vi "Teleop.vi"(10 "Match Info":T1={"Autonomous Elapsed Seconds"=0.0, "TeleOp Elapsed Seconds"=0.0, "Disabled Elapsed Seconds"=0.0, "Visited Autonomous"=FALSE, "Visited TeleOp"=FALSE, "Visited Disabled"=FALSE, "Autonomous Settings"={"Autonomous Style"=enum."Independent", "VI Refnum"=refnum}}, 11 "Call Context":T2) -> ()   [LabVIEW 2019]
doc: "This VI is called for each TeleOp packet received from the DS where the robot is not disabled. It is often used to read from the joysticks and update I/O or to update setpoints for timed control loops. It should complete and return within 20 milliseconds or it may miss DS packets."
uses:
  <vilib>/Rock Robotics/WPI/DriverStation/WPI_DriverStationDerivedRobotMode.ctl
  <vilib>/Rock Robotics/WPI/DriverStation/WPI_DriverStationMatch Info.ctl
  <vilib>/Rock Robotics/WPI/ThirdParty/Phoenix-LabVIEW/Motor Controller/Controls/CTRE_Phoenix_MotorControl_ControlMode.ctl
  <vilib>/Rock Robotics/WPI/Utilities/WPI_GetSetVariantRefNum.vi
  <vilib>/Rock Robotics/WPI/ThirdParty/Phoenix-LabVIEW/Motor Controller/Get/CTRE_Phoenix_MotorController_GetSelectedSensorData.vi
  <vilib>/Rock Robotics/WPI/ThirdParty/Phoenix-LabVIEW/Motor Controller/Get/CTRE_Phoenix_MotorController_GetSupplyAndStatorCurrent_Enhanced.vi
  <vilib>/Rock Robotics/WPI/ThirdParty/Phoenix-LabVIEW/Motor Controller/Get/CTRE_Phoenix_MotorController_GetVoltage.vi
  <vilib>/Rock Robotics/WPI/ThirdParty/Phoenix-LabVIEW/Motor Controller/Get/CTRE_Phoenix_MotorController_IntegratedSensorData_TalonFX.vi
panel:
  out "Waveform Chart":cluster{dbl, "Velocity":dbl}(graph)
  out "RPM":dbl
  out "Velocity (Raw Sensor Units per 100 ms)":i32
  out "Stator Current":dbl
  out "Supply Current":dbl
  out "Joystick Y axis":dbl
  in  "Reverse Peak Percent Output":dbl=-1.0
  in  "Forward Peak Percent Output":dbl=1.0
  out "Output Voltage":dbl
  out "Absolute Position":dbl
  out "Percent Voltage":dbl
  out "Velocity":dbl format="%.2f"
  out "Position":dbl
  # "INFORMATION"
  # "CONTROLS"
  # "FALCON 500 INFORMATION AND CONTROLS"
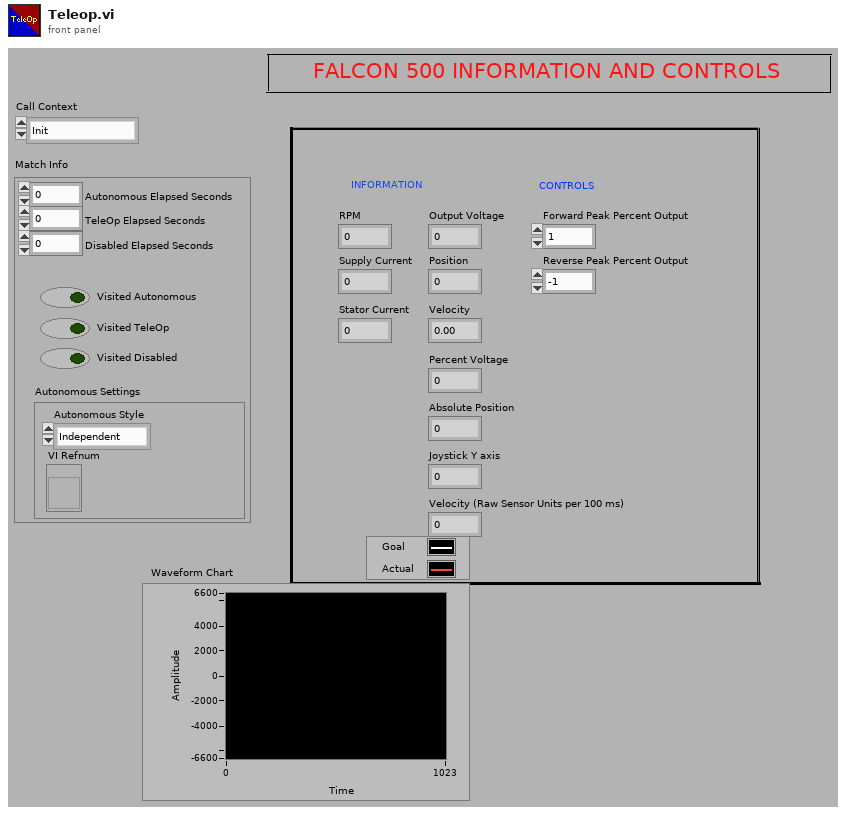
[diagram p1: front panel]
types:
  T1 = typedef "WPI_DriverStationMatch Info.ctl" = cluster{"Autonomous Elapsed Seconds":dbl, "TeleOp Elapsed Seconds":dbl, "Disabled Elapsed Seconds":dbl, "Visited Autonomous":bool, "Visited TeleOp":bool, "Visited Disabled":bool, "Autonomous Settings":cluster{"Autonomous Style":enum16{"Iterative", "Independent"}, "VI Refnum":refnum<vi>}}
  T2 = typedef "WPI_DriverStationDerivedRobotMode.ctl" = enum16{"Init", "Execute", "Stop"}
  T3 = typedef "CTRE_Phoenix_MotorControl_ControlMode.ctl" = u16
  T4 = typedef "WPI_JoystickDevRef.ctl" = cluster{"Device":T5}
  T5 = typedef "WPI_JoystickDeviceEnum.ctl" = enum16{"USB 0", "USB 1", "USB 2", "USB 3", "USB 4", "USB 5"}
  T6 = typedef "WPI_MotorControlDeviceRef.ctl" = cluster{"DeviceStatus":errorcluster, "Type":T7, "PWM":cluster{"PWM Channel":T8, "DeadBand":T9}, "CAN":cluster{"Device Number":u8, "SetOutput VI Ref":variant, "GetOutput VI Ref":variant, "Enable VI Ref":variant, "Disable VI Ref":variant, "Data":variant}, "Invert":bool, "DIO PWM":cluster{"PWM \"Enable\" Channel":T8, "DIOChannel":T10, "PWM Rate":dbl}}
  T7 = typedef "WPI_MotorControlType.ctl" = enum16{"PWM", "CAN", "DIO PWM"}
  T8 = typedef "FPGA_DIOPWMChannel.ctl" = enum8{"PWM 0", "PWM 1", "PWM 2", "PWM 3", "PWM 4", "PWM 5", "PWM 6", "PWM 7", "PWM 8", "PWM 9", "PWM MXP 0", "PWM MXP 1", "PWM MXP 2", "PWM MXP 3", "PWM MXP 4", "PWM MXP 5", "PWM MXP 6", "PWM MXP 7", "PWM MXP 8", "PWM MXP 9", "Invalid"}
  T9 = typedef "WPI_PWMDeadband.ctl" = cluster{"Name":string, "maxPositivePwm":i32, "minPositivePwm":i32, "centerPwm":i32, "maxNegativePwm":i32, "minNegativePwm":i32, "angularRange":u16}
  T10 = typedef "FPGA_DIOChannel.ctl" = enum8{"DIO 0", "DIO 1", "DIO 2", "DIO 3", "DIO 4", "DIO 5", "DIO 6", "DIO 7", "DIO 8", "DIO 9", "DIO MXP 0", "DIO MXP 1", "DIO MXP 2", "DIO MXP 3", "DIO MXP 4", "DIO MXP 5", "DIO MXP 6", "DIO MXP 7", "DIO MXP 8", "DIO MXP 9", "DIO MXP 10", "DIO MXP 11", "DIO MXP 12", "DIO MXP 13", "DIO MXP 14", "DIO MXP 15", "SPI Port CS1", "SPI Port CS2", "SPI Port CS3", "SPI Port MISO", "SPI Port MOSI", "Invalid"}
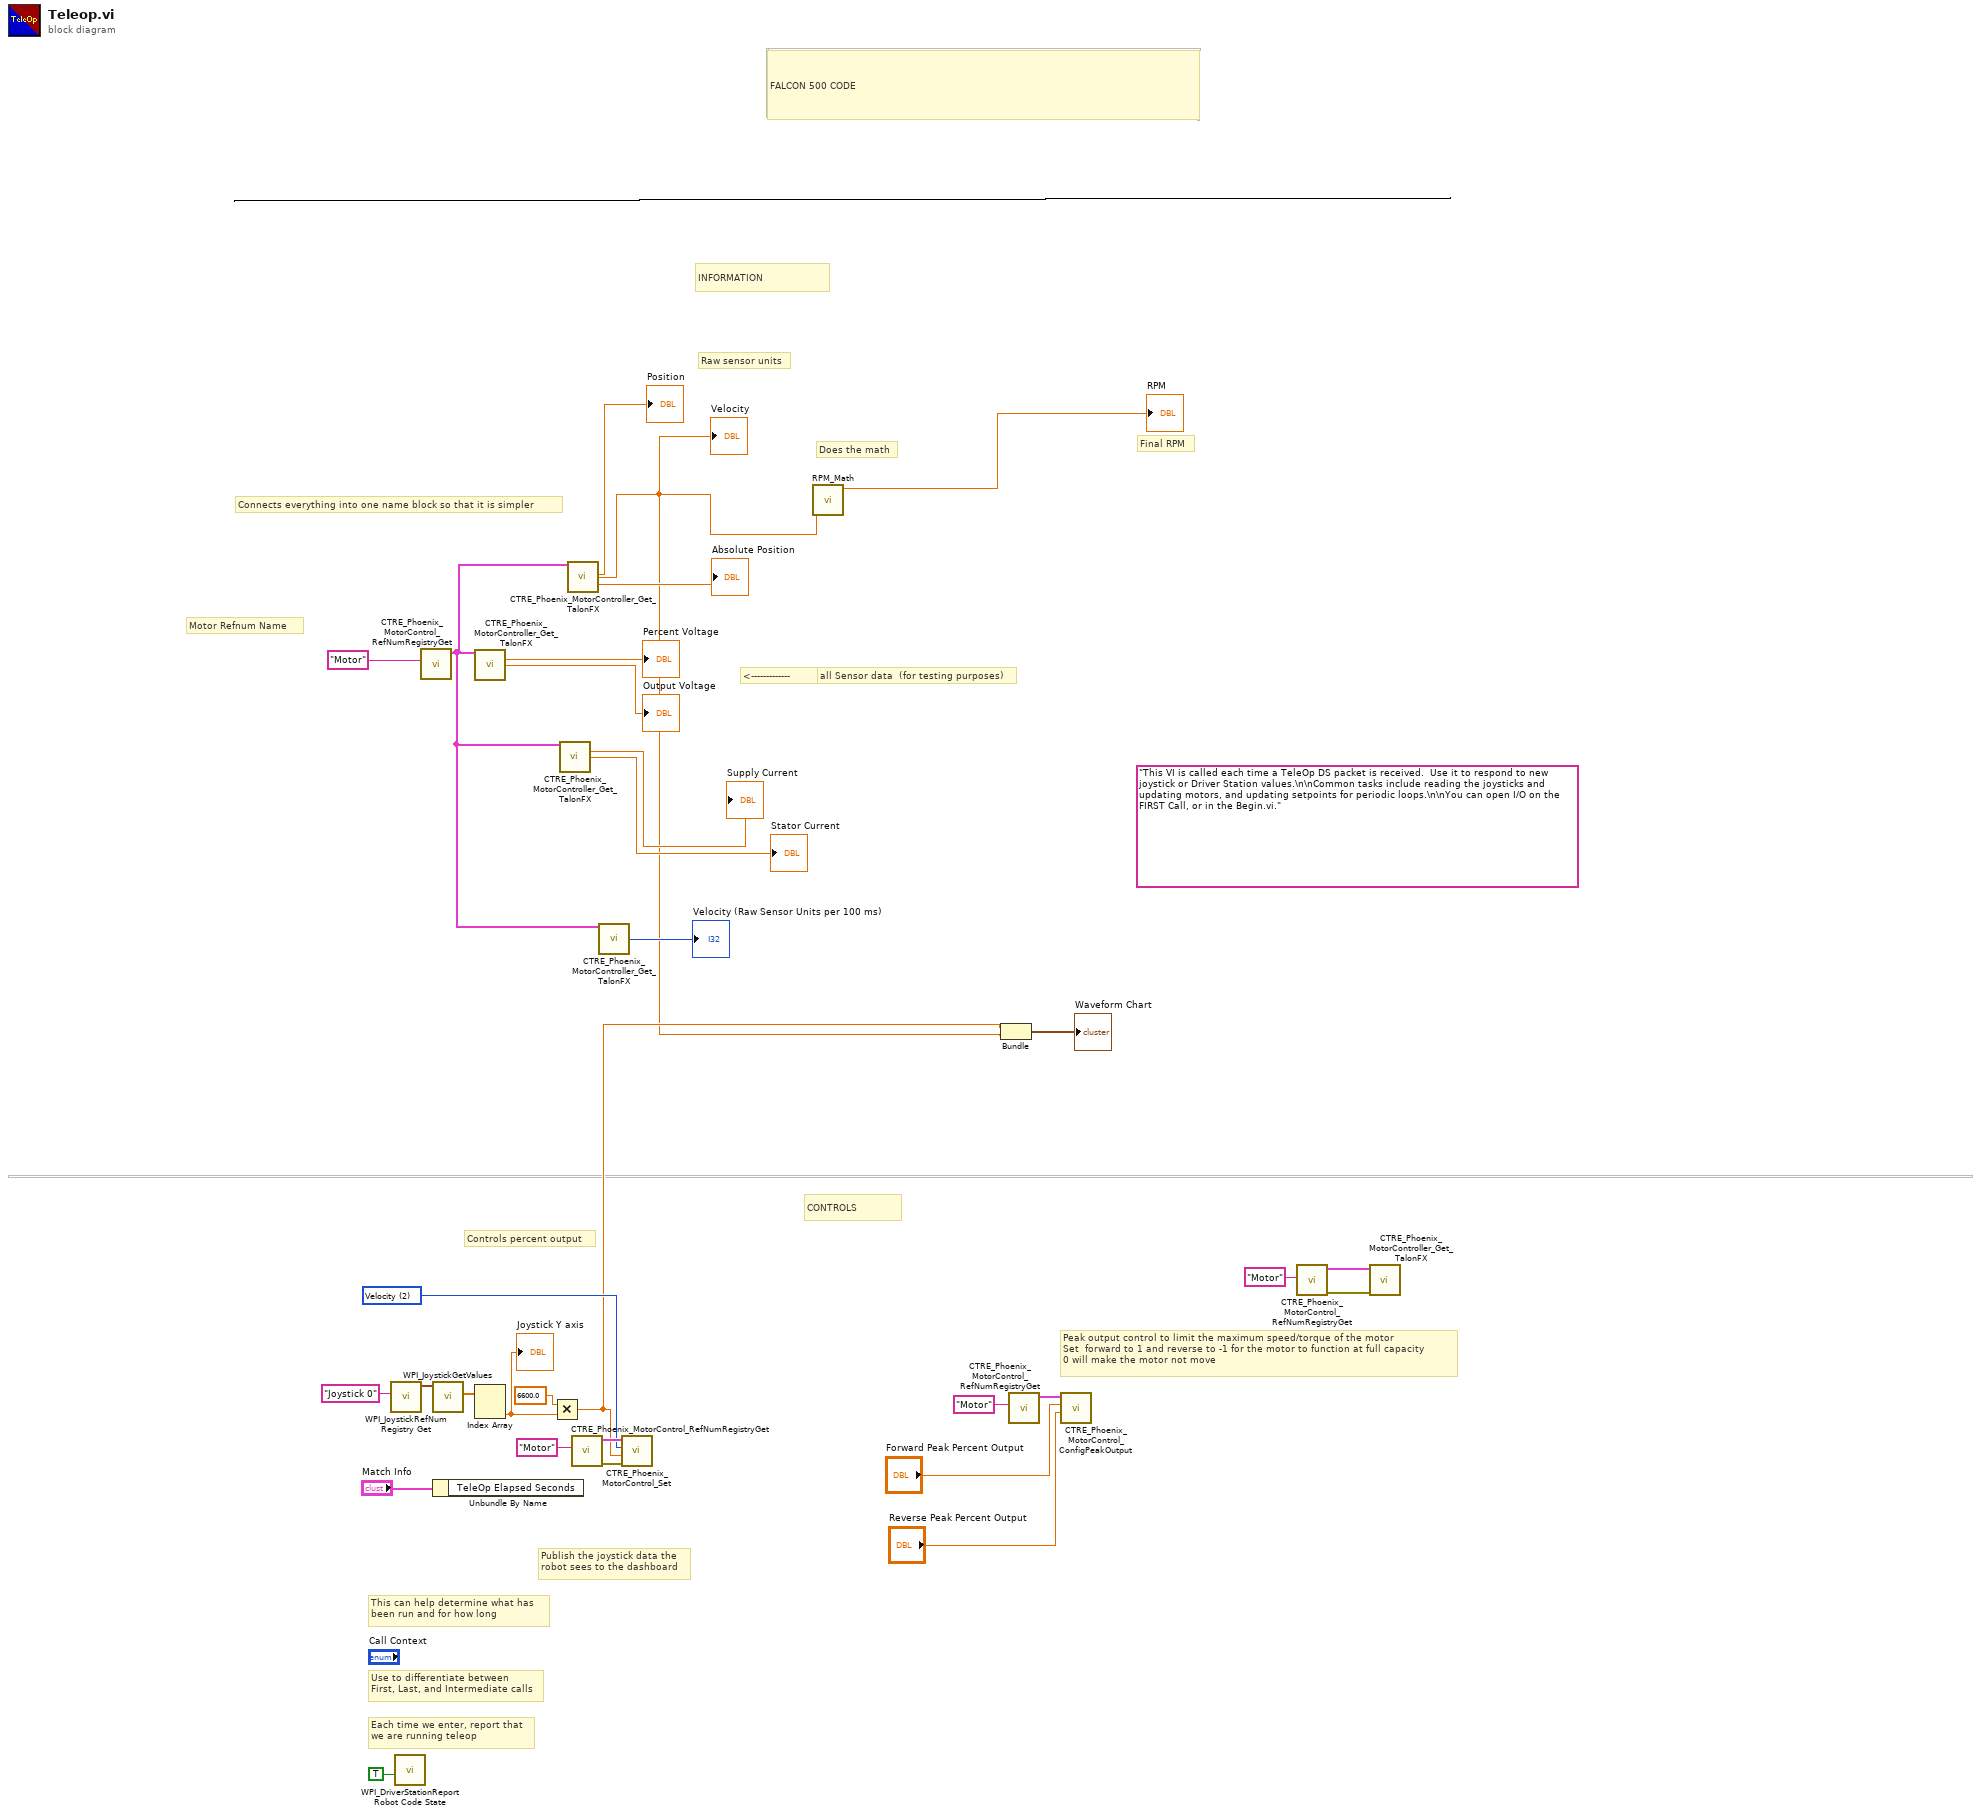
[diagram p0: block diagram]
diagram:
  w16 = T3 2 items=["PercentOutput"=0, "Position"=1, "Velocity"=2, "Current"=3, "Follower"=5, "MotionProfile"=6, "MotionMagic"=7, "MotionProfileArc"=10, "Disabled"=15] ("Control Mode")
  (unwired) "This VI is called each time a TeleOp DS packet is received.  Use it to respond to new joystick or Driver Station values.\n\nCommon tasks include reading the joysticks and updating motors, and updating setpoints for periodic loops.\n\nYou can open I/O on the FIRST Call, or in the Begin.vi."
  # "Final RPM"
  # "Raw sensor units"
  # "INFORMATION"
  # "CONTROLS"
  # "Connects everything into one name block so that it is simpler"
  # "Does the math"
  # "Controls percent output"
  # "<-------------"
  # "Peak output control to limit the maximum speed/torque of the motor\nSet  forward to 1 and reverse to -1 for the motor to function at full capacity\n0 will make the motor not move"
  # "all Sensor data  (for testing purposes)"
  # "FALCON 500 CODE"
  # "Motor Refnum Name"
  # "Publish the joystick data the\nrobot sees to the dashboard"
  # "Each time we enter, report that\nwe are running teleop"
  # "Use to differentiate between\nFirst, Last, and Intermediate calls"
  # "This can help determine what has\nbeen run and for how long"
  n1 = call <vilib>:"WPI_JoystickRefNum Registry Get.vi"("refnum name"="Joystick 0") -> ("JoystickDevRef"=w29:T4)  [unwired: 1 in, 9 out]
  n2 = call <vilib>:"WPI_DriverStationReport Robot Code State.vi"("TeleOp"=TRUE ("Autonomous")) -> ()  [unwired: 10 in, 1 out]
  n3 = call <vilib>:"CTRE_Phoenix_MotorControl_RefNumRegistryGet.vi"("refnum name"="Motor") -> ("PhoenixMotorControlDevRef"=w6:T6)  [unwired: 9 in, 1 out]
  n4 = call <vilib>:"WPI_JoystickGetValues.vi"("JoystickDevRef"=w29) -> ("Axes"=w27:dbl[])  [unwired: 6 in, 4 out]
  n5 = Unbundle By Name("Match Info") -> ()  [unwired: 1 out]
  n6 = call-poly <vilib>:"CTRE_Phoenix_MotorController_Get_TalonFX.vi"("PhoenixMotorControlDevRef"=w6) -> ("Percent Output"=→"Percent Voltage":dbl, "Output Voltage"=→"Output Voltage":dbl)  [unwired: 10 in, 3 out]
  n7 = Index Array(array=w27) -> (element #2=w4:dbl)  [unwired: 2 in, 1 out]
  "Joystick Y axis" <- w4
  n8 = Multiply(x=6600.0, y=w4) -> (x*y=w3:dbl)
  n9 = call-poly <vilib>:"CTRE_Phoenix_MotorController_Get_TalonFX.vi"("PhoenixMotorControlDevRef"=w6) -> ("Supply Current"=→"Supply Current":dbl, "Stator Current"=→"Stator Current":dbl)  [unwired: 11 in, 2 out]
  n10 = call-poly <vilib>:"CTRE_Phoenix_MotorController_Get_TalonFX.vi"("PhoenixMotorControlDevRef"=w6) -> ("Position"=→"Position":dbl, "Velocity"=w2:dbl, "Absolute Position"=→"Absolute Position":dbl)  [unwired: 10 in, 2 out]
  "Velocity" <- w2
  n11 = call <vilib>:"CTRE_Phoenix_MotorControl_RefNumRegistryGet.vi"("refnum name"="Motor") -> ("error out"=w15:errorcluster, "PhoenixMotorControlDevRef"=w17:T6)  [unwired: 9 in]
  n12 = call-poly <vilib>:"CTRE_Phoenix_MotorController_Get_TalonFX.vi"("PhoenixMotorControlDevRef"=w6) -> ("Velocity (Raw Sensor Units per 100 ms)"=→"Velocity (Raw Sensor Units per 100 ms)":i32)  [unwired: 11 in, 3 out]
  n13 = call <vilib>:"CTRE_Phoenix_MotorControl_Set.vi"("error in (no error)"=w15, "Output"=w3, "Control Mode"=w16, "PhoenixMotorControlDevRef"=w17) -> ()  [unwired: 6 in, 2 out]
  n14 = call "RPM_Math.vi"("Velocity in"=w2) -> ("RPM"=→"RPM":dbl)  [unwired: 10 in]
  n15 = Bundle(w3, "Velocity"=w2) -> (→"Waveform Chart":cluster{dbl, "Velocity":dbl})  [unwired: 1 in]
  n16 = call <vilib>:"CTRE_Phoenix_MotorControl_RefNumRegistryGet.vi"("refnum name"="Motor") -> ("PhoenixMotorControlDevRef"=w19:T6)  [unwired: 9 in, 1 out]
  n17 = call <vilib>:"CTRE_Phoenix_MotorControl_ConfigPeakOutput.vi"("Reverse Peak Percent Output"="Reverse Peak Percent Output", "Forward Peak Percent Output"="Forward Peak Percent Output", "PhoenixMotorControlDevRef"=w19) -> ()  [unwired: 7 in, 2 out]
  n18 = call <vilib>:"CTRE_Phoenix_MotorControl_RefNumRegistryGet.vi"("refnum name"="Motor") -> ("error out"=w7:errorcluster, "PhoenixMotorControlDevRef"=w8:T6)  [unwired: 9 in]
  n19 = call-poly <vilib>:"CTRE_Phoenix_MotorController_Get_TalonFX.vi"("PhoenixMotorControlDevRef"=w8, "error in"=w7) -> ()  [unwired: 9 in, 5 out]
